vi "Activate Process Tree View.vi"(8 "error in (no error)":errorcluster, 11 "Main In":refnum<class "Main.lvclass">) -> (0 "error out":errorcluster, 2 "VI Ref":refnum<vi>, 3 "Main Out":refnum<class "Main.lvclass">)   [LabVIEW 2020, in "Main.lvclass"]
uses:
  Main.lvclass
  Process Tree View/Process Tree View.lvclass
  C:/Users/anton/Documents/GitHub/triarc-debugger/source/Debug View/Debug View.lvclass
  Debug View/Debug View.lvclass/Debug View.ctl
  Debugger/Debugger.lvclass
  C:/Users/anton/Documents/GitHub/triarc-debugger/source/Process/Debug Process.lvclass
  Main.lvclass/Main.ctl
  Debug View/Debug View.lvclass
  C:/Users/anton/Documents/GitHub/triarc-debugger/source/Process Tree View/Process Tree View.lvclass
  Process Tree View Model/Process Tree View Model.lvclass
  C:/Users/anton/Documents/GitHub/triarc-debugger/source/Debugger/Debugger.lvclass
  C:/Users/anton/Documents/GitHub/triarc-debugger/source/Debug Data Event/Debug Data Listener.lvclass
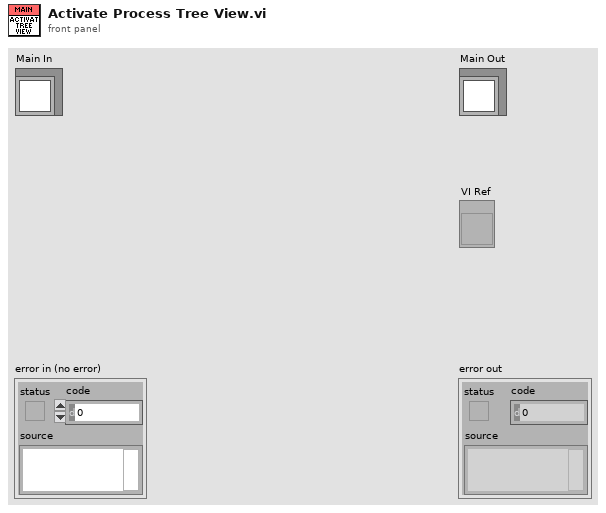
[diagram p1: front panel]
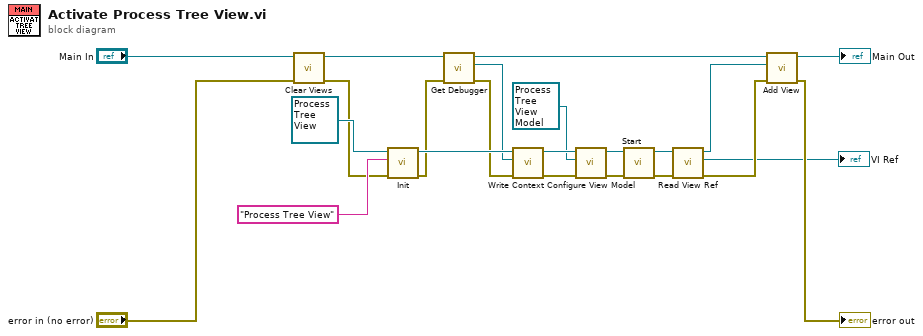
[diagram p0: block diagram]
diagram:
  n1 = call "Clear Views.vi"("error in (no error)"="error in (no error)", "Main In"="Main In") -> ("error out"=w5:errorcluster, "Main Out"=w20:refnum<class "Main.lvclass">)  [unwired: 8 in]
  n2 = call-dynamic "Init.vi"("error in (no error)"=w5, "Name"="Process Tree View", "Debug View In"=refnum<class "Process Tree View.lvclass"> refnum ("Process Tree View.lvclass")) -> ("error out"=w18:errorcluster, "Debug View Out"=w21:refnum<class "Process Tree View.lvclass">)  [unwired: 7 in]
  n3 = call "Get Debugger.vi"("error in (no error)"=w18, "Main In"=w20) -> ("error out"=w17:errorcluster, "Debugger.lvclass"=w19:refnum<class "Debugger.lvclass">, "Main Out"=w13:refnum<class "Main.lvclass">)  [unwired: 7 in]
  n4 = call "Write Context.vi"("error in (no error)"=w17, "Debug Process.lvclass"=w19, "Debug View In"=w21) -> ("error out"=w22:errorcluster, "Debug View Out"=w3:refnum<class "Process Tree View.lvclass">)  [unwired: 7 in]
  n5 = call "Configure View Model.vi"("error in (no error)"=w22, "List Box View Model"=refnum<class "Process Tree View Model.lvclass"> refnum ("Process Tree View Model.lvclass"), "List Box View In"=w3) -> ("error out"=w4:errorcluster, "List Box View Out"=w2:refnum<class "Process Tree View.lvclass">)  [unwired: 7 in]
  n6 = call "Start.vi"("error in (no error)"=w4, "Debug View In"=w2) -> ("error out"=w15:errorcluster, "Debug View Out"=w16:refnum<class "Process Tree View.lvclass">)  [unwired: 8 in]
  n7 = call "Read View Ref.vi"("error in (no error)"=w15, "Debug View In"=w16) -> ("error out"=w14:errorcluster, "View Ref"=→"VI Ref":refnum<vi>, "Debug View Out"=w12:refnum<class "Process Tree View.lvclass">)  [unwired: 7 in]
  n8 = call "Add View.vi"("error in (no error)"=w14, "Debug Process"=w12, "Main In"=w13) -> ("error out"=→"error out":errorcluster, "Main Out"=→"Main Out":refnum<class "Main.lvclass">)  [unwired: 7 in]
